vi "ClosePSOC.vi"(8 "error in":errorcluster, 11 "VISA resource name":refnum<visa-resource-name>="COM1") -> (0 "error out":errorcluster)   [LabVIEW 2012]
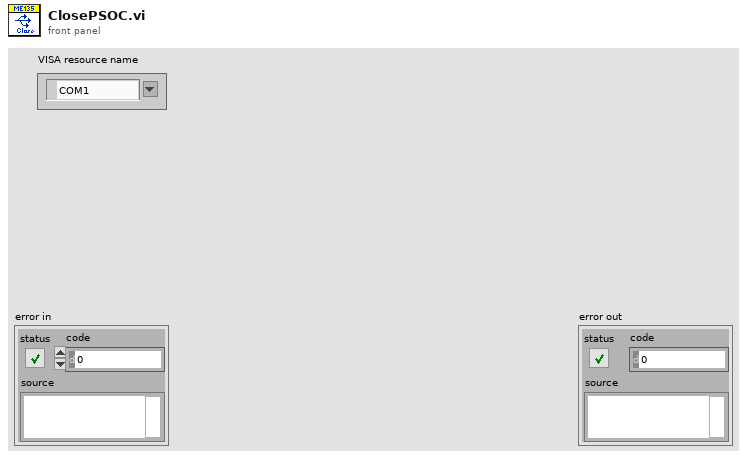
[diagram p1: front panel]
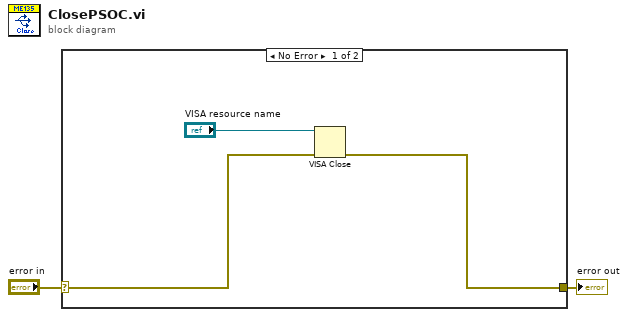
[diagram p0: block diagram]
diagram:
  n1 = case shown="No Error" "error in" {
    selector: "error in" -> [w4 w6]
    tunnel: [w3 w6] -> w1
    frame No Error {
      n2 = VISA Close(VISA resource name="VISA resource name", error in (no error)=w4) -> (error out=w3:errorcluster)
    }
    frame Error {
    }
  }
  "error out" <- w1
